vi "fgvTcpQueueRx.vi"(8 "Error In":errorcluster caption="에러 입력", 10 "Write":string, 11 "Function":T1) -> (0 "Error Out":errorcluster caption="에러 출력", 2 "Read":string, 3 "Count":i32)   [LabVIEW 2018]
uses:
  control/enumFgvFunction.ctl
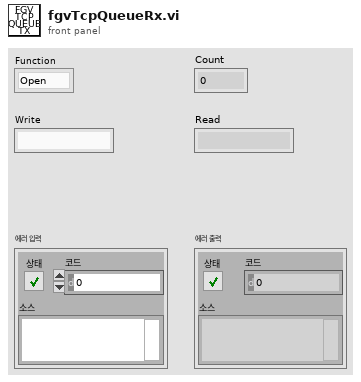
[diagram p1: front panel]
types:
  T1 = typedef "enumFgvFunction.ctl" = enum16{"Open", "Read", "Check", "Write", "Close"}
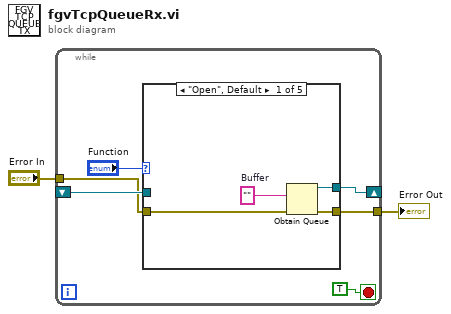
[diagram p0: block diagram]
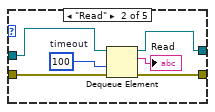
[diagram p2: hidden frame]
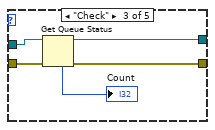
[diagram p3: hidden frame]
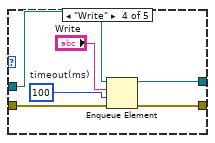
[diagram p4: hidden frame]
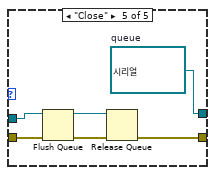
[diagram p5: hidden frame]
diagram:
  n1 = while {
    shift-right: [w6] -> _
    shift-left: _ -> [w7]
    tunnel: "Error In" -> [w5]
    tunnel: [w4] -> w1
    stop <- TRUE stop-if-true
    n2 = case shown="\"Open\", Default" "Function" {
      tunnel: w7 -> [_ w18 w23 w29 w35]
      tunnel: [w12 w17 w22 w28 w33] -> w6
      tunnel: w5 -> [w9 w15 w20 w26 w32]
      tunnel: [w10 w14 w19 w25 w30] -> w4
      frame "Open", Default {
        w11 = ""  # Buffer
        n3 = Obtain Queue(element data type=w11, error in (no error)=w9) -> (queue out=w12:refnum<queue>, error out=w10:errorcluster)  [unwired: 3 in, 1 out]
      }
      frame "Read" {
        w13 = 100  # timeout
        n4 = Dequeue Element(queue=w18, timeout in ms (-1)=w13, error in (no error)=w15) -> (queue out=w17:refnum<queue>, element=→"Read":string, error out=w14:errorcluster)  [unwired: 1 out]
      }
      frame "Check" {
        n5 = Get Queue Status(queue=w23, error in (no error)=w20) -> (queue out=w22:refnum<queue>, error out=w19:errorcluster, # elements in queue=→"Count":i32)  [unwired: 1 in, 5 out]
      }
      frame "Write" {
        w24 = 100  # timeout(ms)
        n6 = Enqueue Element(queue=w29, element="Write", timeout in ms (-1)=w24, error in (no error)=w26) -> (queue out=w28:refnum<queue>, error out=w25:errorcluster)  [unwired: 1 out]
      }
      frame "Close" {
        w33 = refnum<queue> refnum  # queue
        n7 = Flush Queue(queue=w35, error in (no error)=w32) -> (queue out=w34:refnum<queue>, error out=w31:errorcluster)  [unwired: 1 out]
        n8 = Release Queue(queue=w34, error in (no error)=w31) -> (error out=w30:errorcluster)  [unwired: 1 in, 2 out]
      }
    }
  }
  "Error Out" <- w1
